vi "RH_PPMU_Configure.vi"(7 "Digital_Parameters":T2, 8 "error in":errorcluster, 9 "output function":T1=1300 items=["DC Voltage"=1300, "DC Current"=1301], 10 "channel list":string, 11 "PPMU Session In":refnum<k15>) -> (0 "error out":errorcluster, 3 "PPMU Session Out":refnum<k15>)   [LabVIEW 2023, in "ResourceHandling.lvlib"]
doc: "Configures PPMU channels in Voltage or Current mode as well as the Aperture Time"
uses:
  ResourceHandling.lvlib
  TypeDefs/RH_PPMU_Parameters.ctl
  <instrlib>/niDigital/niDigital.llb/niDigital Output Function.ctl
  <instrlib>/niDigital/niDigital.llb/niDigital Selected Function.ctl
  <instrlib>/niDigital/niDigital.llb/niDigital PMU Aperture Time Units.ctl
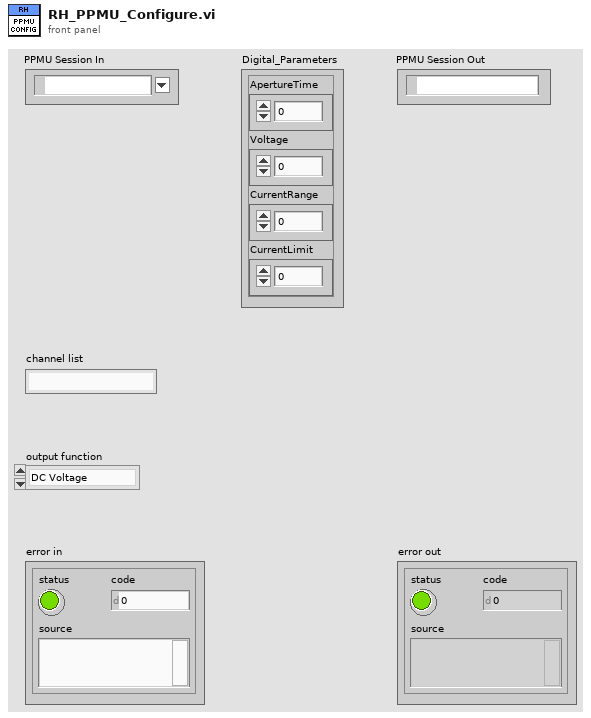
[diagram p1: front panel]
types:
  T1 = typedef "niDigital Output Function.ctl" = i32
  T2 = typedef "ResourceHandling.lvlib/RH_PPMU_Parameters.ctl" = cluster{"ApertureTime":dbl, "Voltage":dbl, "CurrentRange":dbl, "CurrentLimit":dbl}
  T3 = typedef "niDigital PMU Aperture Time Units.ctl" = i32
  T4 = typedef "niDigital Selected Function.ctl" = i32
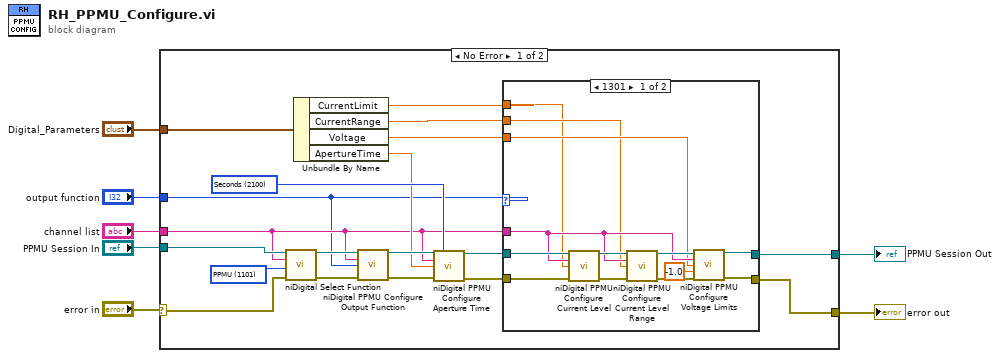
[diagram p0: block diagram]
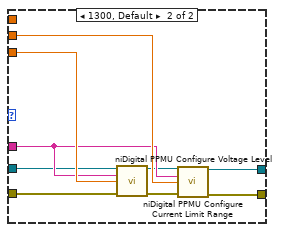
[diagram p2: hidden frame]
diagram:
  n1 = case shown="No Error" "error in" {
    selector: "error in" -> [w8 w50]
    tunnel: "PPMU Session In" -> [w26 w49]
    tunnel: "Digital_Parameters" -> [w19 _]
    tunnel: "channel list" -> [w15 _]
    tunnel: [w13 w50] -> w2
    tunnel: [w12 w49] -> w4
    tunnel: "output function" -> [w9 _]
    frame No Error {
      w20 = T3 2100 items=["Seconds"=2100] ("aperture time units")
      w25 = T4 1101 items=["Digital"=1100, "PPMU"=1101, "Off"=1102, "Disconnect"=1103] ("function")
      n2 = call <instrlib>:"niDigital Select Function.vi"("instrument handle"=w26, "channel list"=w15, "function"=w25, "error in"=w8) -> ("instrument handle out"=w24:refnum<k15>, "error out"=w23:errorcluster)  [unwired: 10 in]
      n3 = Unbundle By Name(w19) -> ("CurrentLimit"=w14:dbl, "CurrentRange"=w16:dbl, "Voltage"=w17:dbl, "ApertureTime"=w18:dbl)
      n4 = call <instrlib>:"niDigital PPMU Configure Output Function.vi"("instrument handle"=w24, "channel list"=w15, "output function"=w9, "error in"=w23) -> ("instrument handle out"=w22:refnum<k15>, "error out"=w21:errorcluster)  [unwired: 10 in]
      n5 = call <instrlib>:"niDigital PPMU Configure Aperture Time.vi"("instrument handle"=w22, "aperture time units"=w20, "channel list"=w15, "aperture time"=w18, "error in"=w21) -> ("instrument handle out"=w11:refnum<k15>, "error out"=w10:errorcluster)  [unwired: 9 in]
      n6 = case shown="1301" w9 {
        tunnel: w17 -> [w29 w48]
        tunnel: w16 -> [w28 w47]
        tunnel: w15 -> [w31 w46]
        tunnel: w14 -> [w27 _]
        tunnel: [w33 w40] -> w13
        tunnel: [w32 w41] -> w12
        tunnel: w11 -> [w39 w45]
        tunnel: w10 -> [w38 w44]
        frame 1301 {
          n7 = call <instrlib>:"niDigital PPMU Configure Current Level.vi"("instrument handle"=w39, "channel list"=w31, "current level (A)"=w27, "error in"=w38) -> ("instrument handle out"=w37:refnum<k15>, "error out"=w36:errorcluster)  [unwired: 10 in]
          n8 = call <instrlib>:"niDigital PPMU Configure Current Level Range.vi"("instrument handle"=w37, "channel list"=w31, "current level range (A)"=w28, "error in"=w36) -> ("instrument handle out"=w35:refnum<k15>, "error out"=w34:errorcluster)  [unwired: 10 in]
          n9 = call <instrlib>:"niDigital PPMU Configure Voltage Limits.vi"("instrument handle"=w35, "channel list"=w31, "voltage limit high (V)"=w29, "voltage limit low (V)"=-1.0, "error in"=w34) -> ("instrument handle out"=w32:refnum<k15>, "error out"=w33:errorcluster)  [unwired: 9 in]
        }
        frame 1300, Default {
          n10 = call <instrlib>:"niDigital PPMU Configure Voltage Level.vi"("instrument handle"=w45, "channel list"=w46, "voltage level (V)"=w48, "error in"=w44) -> ("instrument handle out"=w42:refnum<k15>, "error out"=w43:errorcluster)  [unwired: 10 in]
          n11 = call <instrlib>:"niDigital PPMU Configure Current Limit Range.vi"("instrument handle"=w42, "channel list"=w46, "current limit range (A)"=w47, "error in"=w43) -> ("instrument handle out"=w41:refnum<k15>, "error out"=w40:errorcluster)  [unwired: 10 in]
        }
      }
    }
    frame Error {
    }
  }
  "PPMU Session Out" <- w4
  "error out" <- w2
